vi "Testing - Update ATM Messages.vi"(8 "error in":errorcluster) -> (0 "error out":errorcluster)   [LabVIEW 2020, in "ATM.lvlib"]
doc: "_____\nCreated using DQMH Framework: Event Scripter 7.1.0.1503."
uses:
  ATM.lvlib
  Testing - Update ATM Messages Argument--cluster.ctl
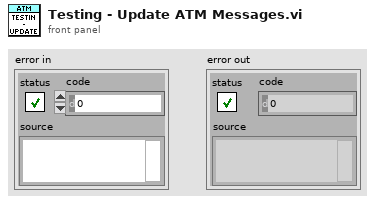
[diagram p1: front panel]
types:
  T1 = typedef "ATM.lvlib/Testing - Update ATM Messages Argument--cluster.ctl" = cluster{"Boolean":bool}
  T2 = typedef "ATM.lvlib/Request Events--cluster.ctl" = cluster{"Stop Module":refnum<user-event>, "Show Panel":refnum<user-event>, "Hide Panel":refnum<user-event>, "Get Module Execution Status":refnum<user-event>, "Show Diagram":refnum<user-event>, "Private.Set Up Controls":refnum<user-event>, "Private.Update ATM Messages":refnum<user-event>, "Private.Start Timeout":refnum<user-event>, "Private.Set Up Accounts File":refnum<user-event>, "Private.Verification OK":refnum<user-event>, "Private.Session Timed Out":refnum<user-event>, "Private.Verification NOK":refnum<user-event>, "Private.Stop Timeout":refnum<user-event>, "Private.Deposit Introduced":refnum<user-event>, "Private.Save Account":refnum<user-event>, "Private.Check Withdrawal":refnum<user-event>, "Testing - Update ATM Messages":refnum<user-event>, "Testing - Generate File Not Found Error":refnum<user-event>, "Testing - Enable All Elements in FP":refnum<user-event>, "Testing - Disable All Elements in FP":refnum<user-event>}
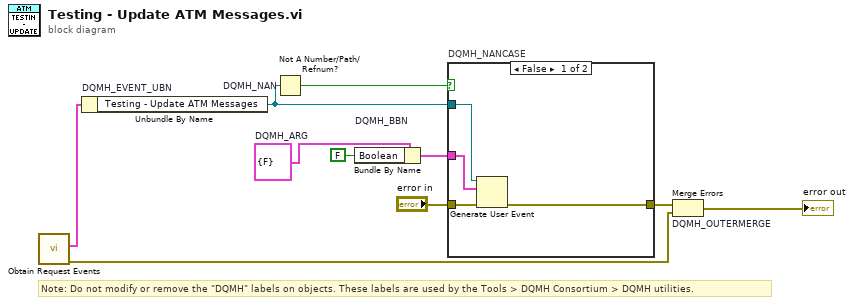
[diagram p0: block diagram]
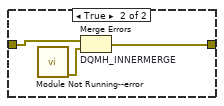
[diagram p2: hidden frame]
diagram:
  w4 = T1 {"Boolean"=FALSE}  # DQMH_ARG
  # "Note: Do not modify or remove the \"DQMH\" labels on objects. These labels are used by the Tools > DQMH Consortium > DQMH utilities."
  n1 = call "Obtain Request Events.vi"() -> ("error out"=w3:errorcluster, "ATM Request Events"=w2:T2)  [unwired: 10 in]
  n2 = Unbundle By Name "DQMH_EVENT_UBN"(w2) -> ("Testing - Update ATM Messages"=w6:refnum<user-event>)
  n3 = Not A Number/Path/Refnum? "DQMH_NAN"(number/path/refnum=w6) -> (NaN/Path/Refnum?=w7:bool)
  n4 = Bundle By Name "DQMH_BBN"(cluster=w4, "Boolean"=FALSE) -> (w8:T1)
  n5 = case "DQMH_NANCASE" shown="False" w7 {
    tunnel: "error in" -> [w14 w17]
    tunnel: [w13 w16] -> w5
    tunnel: w6 -> [w12 _]
    tunnel: w8 -> [w11 _]
    frame False {
      n6 = Generate User Event(user event=w12, event data cluster=w11, error in=w14) -> (error out=w13:errorcluster)  [unwired: 1 in, 1 out]
    }
    frame True {
      n7 = call "Module Not Running--error.vi"() -> ("error out"=w15:errorcluster)  [unwired: 11 in]
      n8 = Merge Errors "DQMH_INNERMERGE"(w17, w15) -> (w16:errorcluster)
    }
  }
  n9 = Merge Errors "DQMH_OUTERMERGE"(w5, w3) -> (→"error out":errorcluster)
